vi "MG3700 Header Mode.vi"(4 "Error in (no error)":errorcluster, 5 "Mode (OFF)":T2, 6 "Set/Get (Set)":T1, 7 "VISA In":refnum<visa-resource-name>) -> (0 "Error out":errorcluster, 1 "Error code":i32, 2 "Mode out":T2, 3 "VISA Out":refnum<visa-resource-name>)   [LabVIEW 2015]
doc: "Function: Specifies whether to append (On) a response header or not (Off)."
uses:
  MG3700A/Controls/On_Off.ctl
  MG3700A/Controls/Set_Get.ctl
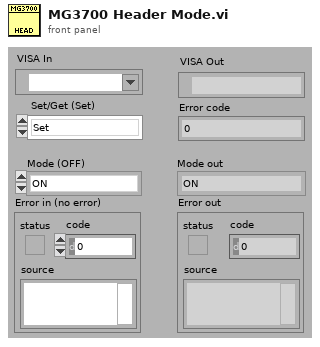
[diagram p1: front panel]
types:
  T1 = typedef "Set_Get.ctl" = enum16{"Set", "Get"}
  T2 = typedef "On_Off.ctl" = enum16{"ON", "OFF"}
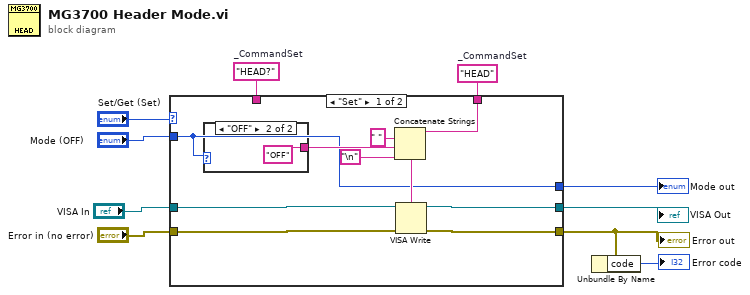
[diagram p0: block diagram]
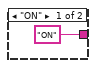
[diagram p2: hidden frame]
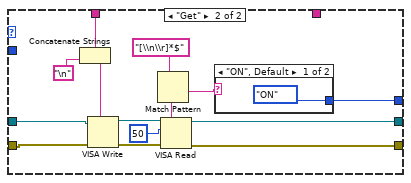
[diagram p3: hidden frame]
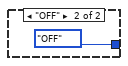
[diagram p4: hidden frame]
diagram:
  w3 = "HEAD?"  # _CommandSet
  w2 = "HEAD"  # _CommandSet
  n1 = case shown="\"Set\"" "Set/Get (Set)" {
    tunnel: "Mode (OFF)" -> [w11 _]
    tunnel: "VISA In" -> [w17 w33]
    tunnel: [w18 w27] -> w8
    tunnel: "Error in (no error)" -> [w16 w25]
    tunnel: [w15 w26] -> w6
    tunnel: [w11 w28] -> w4
    tunnel: w3 -> [_ w36]
    tunnel: w2 -> [w14 _]
    frame "Set" {
      n2 = case shown="\"OFF\"" w11 {
        tunnel: ["ON" "OFF"] -> w19
        frame "ON" {
        }
        frame "OFF" {
        }
      }
      n3 = Concatenate Strings(w14, " " ("Substring"), w19, "\n") -> (w12:string)
      n4 = VISA Write(VISA resource name=w17, write buffer=w12, error in (no error)=w16) -> (VISA resource name out=w18:refnum<visa-resource-name>, error out=w15:errorcluster)  [unwired: 1 out]
    }
    frame "Get" {
      n5 = Concatenate Strings(w36, "\n") -> (w35:string)
      n6 = VISA Write(VISA resource name=w33, write buffer=w35, error in (no error)=w25) -> (VISA resource name out=w32:refnum<visa-resource-name>, error out=w24:errorcluster)  [unwired: 1 out]
      n7 = VISA Read(VISA resource name=w32, byte count=u32 50 ("byte count (0)"), error in (no error)=w24) -> (VISA resource name out=w27:refnum<visa-resource-name>, read buffer=w31:string, error out=w26:errorcluster)  [unwired: 1 out]
      n8 = Match Pattern(string=w31, regular expression="[\\n\\r]*$") -> (after substring=w29:string)  [unwired: 1 in, 3 out]
      n9 = case shown="\"ON\", Default" w29 {
        tunnel: [On_Off."ON" ("Mode (ON)") On_Off."OFF" ("Mode (ON)")] -> w28
        frame "ON", Default {
        }
        frame "OFF" {
        }
      }
    }
  }
  "VISA Out" <- w8
  "Error out" <- w6
  "Mode out" <- w4
  n10 = Unbundle By Name(w6) -> ("code"=→"Error code":i32)
